vi "LSX Get Limit.vi"(7 "pdMaxRange":dbl, 8 "error in (no error)":errorcluster, 9 "pdMinRange":dbl, 10 "lAxis":i32, 11 "lLSID":i32) -> (0 "error out":errorcluster, 1 "pdMinRange out":dbl, 3 "function return":i32, 5 "pdMaxRange out":dbl)   [LabVIEW 2016, in "Tango_DLL.lvlib"]
doc: "TANGOAPI int TANGOCALL LSX_GetLimit (int lLSID, int lAxis, double *pdMinRange, double *pdMaxRange);"
uses:
  Tango_DLL.lvlib
  2017/Microscope Control/Device Library/Stages/Marzhauser/SCAN IM 120 x 80/Tango DLL VIs/Tango_DLL.dll
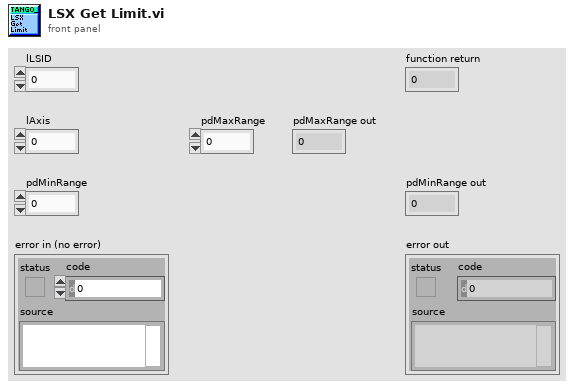
[diagram p1: front panel]
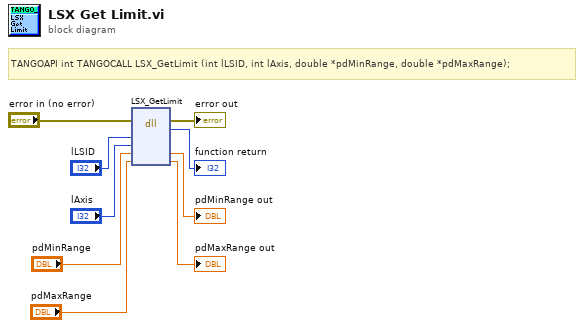
[diagram p0: block diagram]
diagram:
  # "TANGOAPI int TANGOCALL LSX_GetLimit (int lLSID, int lAxis, double *pdMinRange, double *pdMaxRange);"
  n1 = dll-call lib="C:/Users/4PiSMS/Documents/Microscope Control/2017/Microscope Control/Device Library/Stages/Marzhauser/SCAN IM 120 x 80/Tango DLL VIs/Tango_DLL.*" fn="LSX_GetLimit"(error in="error in (no error)", "lLSID"="lLSID", "lAxis"="lAxis", "pdMinRange"="pdMinRange", "pdMaxRange"="pdMaxRange") -> (error out=→"error out":errorcluster, →"function return":i32, "pdMinRange"=→"pdMinRange out":dbl, "pdMaxRange"=→"pdMaxRange out":dbl)  [unwired: 4 in, 1 out]
